vi "Initialization_T_B_ver1.0.vi"(1 "output cluster":T1={"Main Sweep"=0, "Steps Config:"={"total points:"=0, "Step Delay (s)"=0.0, "Ini Delay (s)"=0.0, "# of steps:"=0}, "Temperature Control (ITC 503):"={"GPIB ADR"=0, "Change Heater?"={"Heater?"=FALSE, "Heater"=0}, "Change Temp?"={"Change T?"=FALSE, "Set T (K)"=0.0}, "Cluster"={"Heat Auto?"=FALSE, "Manual Heat?"=FALSE, "Heater (%)"=0.0}, "Change PID?"={"Change PID?"=FALSE, "P"=0.0, "I"=0.0, "D"=0.0}, "Change Para?"=FALSE, "Sensor"=1}, "Temperature Control (LS 340):"={"GPIB ADR"=0, "From (K)"=0.0, "To (K)"=0.0, "Rate (K/min)"=0.0, "Delta T (0.08K)"=0.0, "Temp. Header"="", "T Display Control"={"Ch B"=FALSE, "Ch C"=FALSE, "Ch D"=FALSE}}, "Magnet Control (IPS 120-10)"={"Action"=0, "Standby (s)"=0.0, "Heater on (s)"=0.0, "Sweep Setup "=[], "GPIB ADR"=0, "Change Para?"=FALSE}, "Keithley 6221 :"=[], "Measuring Instruments : "=[], "Lock-In SR7265 :"=[], "Deascription of \nthis measurement"="", "Instruments Config:"=[]} {"Main Sweep" items=["Time", "DC Current", "Delta Current", "Pulse Delta Current", "Sine Current", "Lock-in Vosc"]; "Temperature Control (ITC 503):"."Sensor" items=["T2", "T3"]; "Magnet Control (IPS 120-10)"."Action" items=["Hold", "To Set point", "To Zero", "Clamp"]; "Keithley 6221 :"."Sweep Mode" items=["Linear", "Log", "Exp", "Inverse", "Manual"]}, 5 "Measure with H/T sweep?":bool, 6 "error in (no error)":errorcluster, 7 "First run?":bool, 8 "Last run?":bool, 9 "B Field Display Tex Array":refnum<vi>[](array[refnum]), 10 "Temp. Display Ref Array":refnum<vi>[](array[refnum])) -> (0 "error out":errorcluster, 2 "output cluster 2":T1={"Main Sweep"=0, "Steps Config:"={"total points:"=0, "Step Delay (s)"=0.0, "Ini Delay (s)"=0.0, "# of steps:"=0}, "Temperature Control (ITC 503):"={"GPIB ADR"=0, "Change Heater?"={"Heater?"=FALSE, "Heater"=0}, "Change Temp?"={"Change T?"=FALSE, "Set T (K)"=0.0}, "Cluster"={"Heat Auto?"=FALSE, "Manual Heat?"=FALSE, "Heater (%)"=0.0}, "Change PID?"={"Change PID?"=FALSE, "P"=0.0, "I"=0.0, "D"=0.0}, "Change Para?"=FALSE, "Sensor"=1}, "Temperature Control (LS 340):"={"GPIB ADR"=0, "From (K)"=0.0, "To (K)"=0.0, "Rate (K/min)"=0.0, "Delta T (0.08K)"=0.0, "Temp. Header"="", "T Display Control"={"Ch B"=FALSE, "Ch C"=FALSE, "Ch D"=FALSE}}, "Magnet Control (IPS 120-10)"={"Action"=0, "Standby (s)"=0.0, "Heater on (s)"=0.0, "Sweep Setup "=[], "GPIB ADR"=0, "Change Para?"=FALSE}, "Keithley 6221 :"=[], "Measuring Instruments : "=[], "Lock-In SR7265 :"=[], "Deascription of \nthis measurement"="", "Instruments Config:"=[]} {"Main Sweep" items=["Time", "DC Current", "Delta Current", "Pulse Delta Current", "Sine Current", "Lock-in Vosc"]; "Temperature Control (ITC 503):"."Sensor" items=["T2", "T3"]; "Magnet Control (IPS 120-10)"."Action" items=["Hold", "To Set point", "To Zero", "Clamp"]; "Keithley 6221 :"."Sweep Mode" items=["Linear", "Log", "Exp", "Inverse", "Manual"]}, 3 "Title Array":string[](array[string]), 4 "Comments String":string)   [LabVIEW 2011]
doc: "Initialize the temperature (LS336)"
panel:
  out "BField Display Cluster":cluster{"B":dbl} {"B" min=0.0 format="%_5f"}
  out "B Set Pt (T)":dbl format="%_5g"
  out "B Rate (T/min)":dbl format="%_5g"
  out "Temp Graph 2":dbl[][](graph)=[[348.0650696299951, 348.0650696299951, 348.0650696299951, 348.0650696299951, 348.0650696299951, 348.0650696299951, 348.0650696299951, 348.0650696299951, 348.0650696299951, 348.0650696299951, 348.0650696299951, 348.0650696299951, 348.0650696299951, 348.0650696299951, 348.0650696299951], [349.0, 349.0, 349.0, 349.0, 349.0, 349.0, 349.0, 349.0, 349.0, 349.0, 349.0, 349.0, 349.0, 349.0, 349.0], [347.994, 347.998, 348.007, 348.013, 348.031, 348.047, 348.071, 348.073, 348.076, 348.088, 348.106, 348.11, 348.113, 348.121, 348.128], [349.08, 349.08, 349.08, 349.08, 349.08, 349.08, 349.08, 349.08, 349.08, 349.08, 349.08, 349.08, 349.08, 349.08, 349.08], [348.92, 348.92, 348.92, 348.92, 348.92, 348.92, 348.92, 348.92, 348.92, 348.92, 348.92, 348.92, 348.92, 348.92, 348.92]]
  out "StartTime":u32
  in  "Skip":bool
  out "Time 2":string
  in  "Timeout (min)":u32=30
  out "Reach to set pt?":bool
  out "T Rate (K/min)":dbl format="%_5g"
  out "T Set Pt (K)":dbl format="%_5g"
  out "Temp Display Cluster":cluster{"RMS T:":dbl, "T STD":dbl, "T":dbl} {"T STD" min=0.0 format="%8.4f"; "T" min=0.0 format="%_5f"; "RMS T:" format="%_5g"}
  out "Temp Graph":dbl[][](graph)=[[348.0650696299951, 348.0650696299951, 348.0650696299951, 348.0650696299951, 348.0650696299951, 348.0650696299951, 348.0650696299951, 348.0650696299951, 348.0650696299951, 348.0650696299951, 348.0650696299951, 348.0650696299951, 348.0650696299951, 348.0650696299951, 348.0650696299951], [349.0, 349.0, 349.0, 349.0, 349.0, 349.0, 349.0, 349.0, 349.0, 349.0, 349.0, 349.0, 349.0, 349.0, 349.0], [347.994, 347.998, 348.007, 348.013, 348.031, 348.047, 348.071, 348.073, 348.076, 348.088, 348.106, 348.11, 348.113, 348.121, 348.128], [349.08, 349.08, 349.08, 349.08, 349.08, 349.08, 349.08, 349.08, 349.08, 349.08, 349.08, 349.08, 349.08, 349.08, 349.08], [348.92, 348.92, 348.92, 348.92, 348.92, 348.92, 348.92, 348.92, 348.92, 348.92, 348.92, 348.92, 348.92, 348.92, 348.92]]
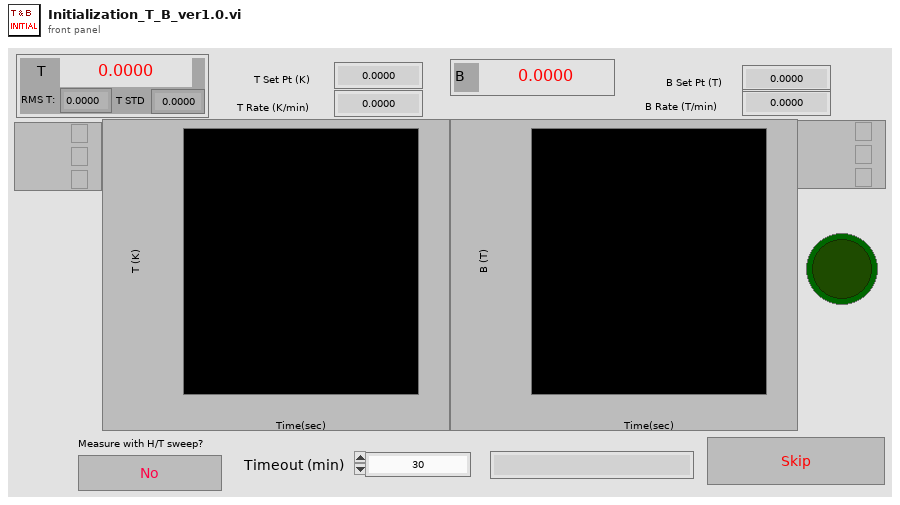
[diagram p1: front panel]
types:
  T1 = cluster{"Main Sweep":u8, "Steps Config:":cluster{"total points:":u32, "Step Delay (s)":dbl, "Ini Delay (s)":dbl, "# of steps:":u32}, "Temperature Control (ITC 503):":cluster{"GPIB ADR":u16, "Change Heater?":cluster{"Heater?":bool, "Heater":u8}, "Change Temp?":cluster{"Change T?":bool, "Set T (K)":dbl}, "Cluster":cluster{"Heat Auto?":bool, "Manual Heat?":bool, "Heater (%)":dbl}, "Change PID?":cluster{"Change PID?":bool, "P":dbl, "I":dbl, "D":dbl}, "Change Para?":bool, "Sensor":u16}, "Temperature Control (LS 340):":cluster{"GPIB ADR":u16, "From (K)":dbl, "To (K)":dbl, "Rate (K/min)":dbl, "Delta T (0.08K)":dbl, "Temp. Header":string, "T Display Control":cluster{"Ch B":bool, "Ch C":bool, "Ch D":bool}}, "Magnet Control (IPS 120-10)":cluster{"Action":u16, "Standby (s)":dbl, "Heater on (s)":dbl, "Sweep Setup ":cluster{"Set Point (T)":dbl, "Set Rate(T/min)":dbl, "Hold(min)":dbl}[], "GPIB ADR":u16, "Change Para?":bool}, "Keithley 6221 :":cluster{"Delta mode":bool, "Const I":bool, "Pulse Delta mode":bool, "Sine Wave Mode":bool, "From I_HI (A)":dbl, "From I (A)":dbl, "I_LO (A)":dbl, "From I_H (A)":dbl, "I_L (A)":dbl, "Freq (Hz)":dbl, "From I_Sin (A)":dbl, "DC Offset (A)":dbl, "Delay Time (s)":dbl, "Pulse Width (s)":dbl, "Delay (s)":dbl, "To I (A)":dbl, "ASymmetric?":bool, "To I_HI (A)":dbl, "To I_H (A)":dbl, "To I_Sin (A)":dbl, "GPIB ADR":u16, "Sweep Mode":u8, "Delta Unit":string, "2182A range (V)":dbl, "6221 Compliance (V)":dbl}[], "Measuring Instruments : ":cluster{"GPIB Bus":dbl, "GPIB Addr":dbl, "Instrument":enum16{"None", "HP34401DMM", "Lockin 7265", "HP3456/7A", "HP3478A", "HP3325FG", "Keithley2182A"}, "Instru Header":string}[], "Lock-In SR7265 :":cluster{"GPIB ADR":u16, "From":dbl, "To":dbl, "Header(;)":string, "Sweep Mode":u8}[], "Deascription of \nthis measurement":string, "Instruments Config:":string[][]}
  T2 = cluster{"GPIB ADR":u16, "Change Heater?":cluster{"Heater?":bool, "Heater":u8}, "Change Temp?":cluster{"Change T?":bool, "Set T (K)":dbl}, "Cluster":cluster{"Heat Auto?":bool, "Manual Heat?":bool, "Heater (%)":dbl}, "Change PID?":cluster{"Change PID?":bool, "P":dbl, "I":dbl, "D":dbl}, "Change Para?":bool, "Sensor":u16}
  T3 = cluster{"GPIB ADR":u16, "From (K)":dbl, "To (K)":dbl, "Rate (K/min)":dbl, "Delta T (0.08K)":dbl, "Temp. Header":string, "T Display Control":cluster{"Ch B":bool, "Ch C":bool, "Ch D":bool}}
  T4 = cluster{"Action":u16, "Standby (s)":dbl, "Heater on (s)":dbl, "Sweep Setup ":cluster{"Set Point (T)":dbl, "Set Rate(T/min)":dbl, "Hold(min)":dbl}[], "GPIB ADR":u16, "Change Para?":bool}
  T5 = cluster{"RMS":dbl, "STD":dbl, "Current value":dbl}
  T6 = cluster{"Com Port":i32, "ISOBUS Address":i32, "GPIB Address":i16, "Communication":enum16{"RS232", "ISOBUS", "GPIB", "Gateway"}}
  T7 = cluster{"GPIB ADR":u16, "Change Heater?":cluster{"Change Heater?":bool, "Heater":u8}, "Change Temp?":cluster{"Change Temp?":bool, "Set Temp (K)":dbl}, "Cluster":cluster{"Heat Auto?":bool, "Manual Heat?":bool, "Heater Manual (%)":dbl}, "Change PID?":cluster{"Change PID?":bool, "Proportional":dbl, "Integral":dbl, "Derivative":dbl}, "Change Para?":bool, "ITC503 Control Sensor":u16}
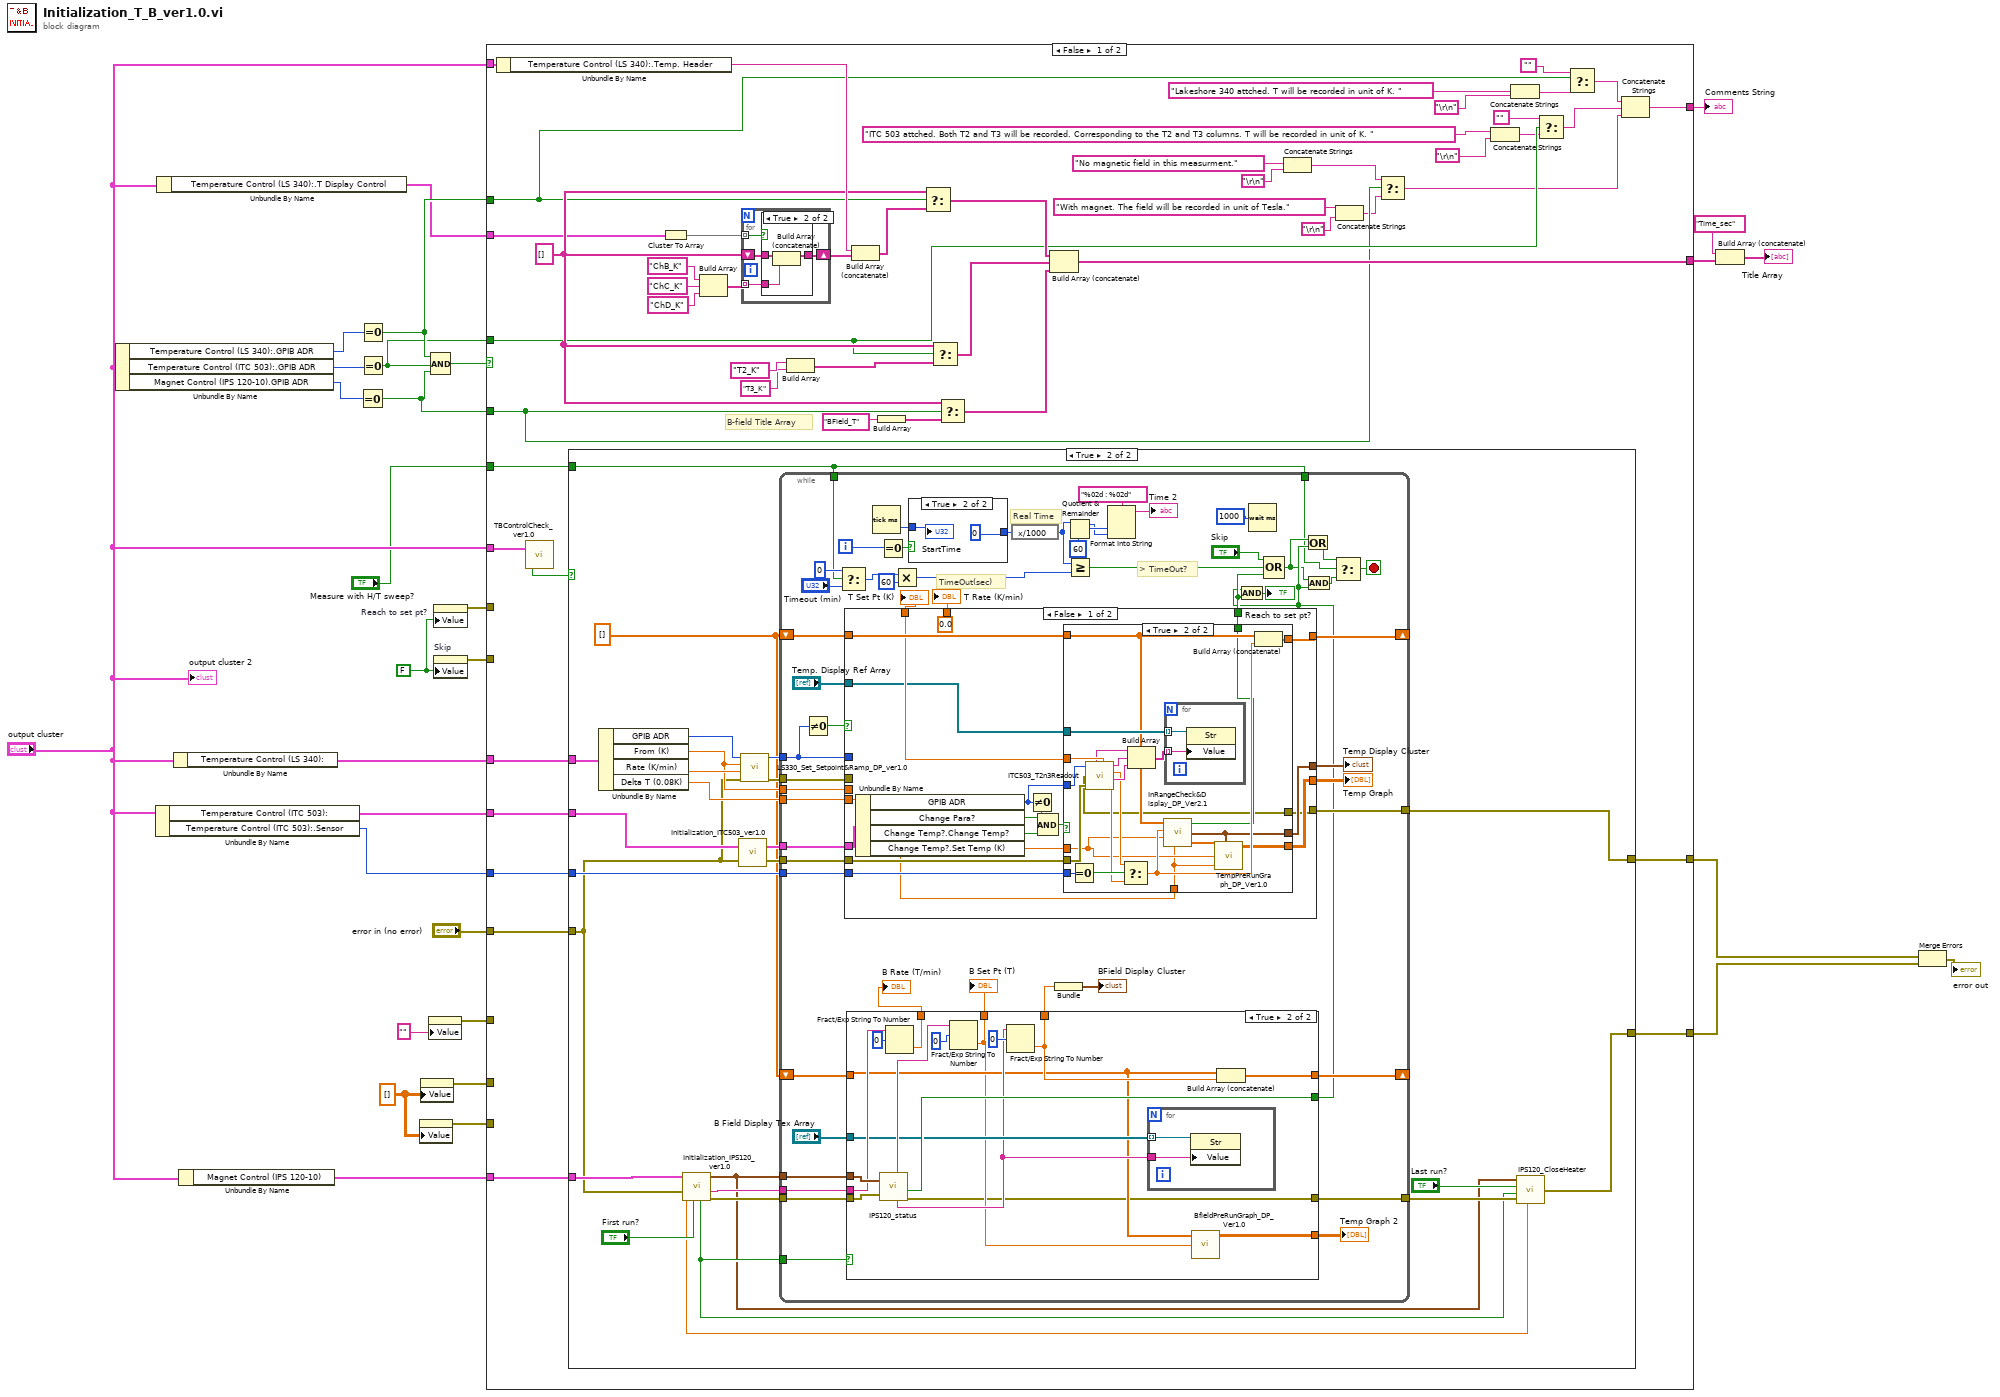
[diagram p0: block diagram]
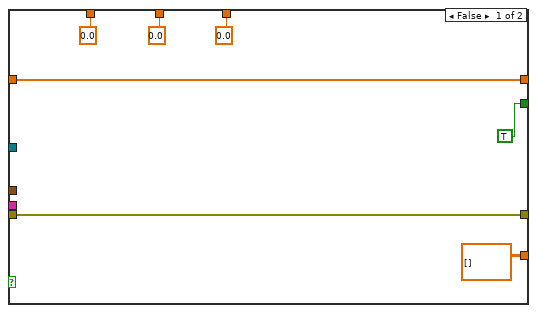
[diagram p3: hidden frame]
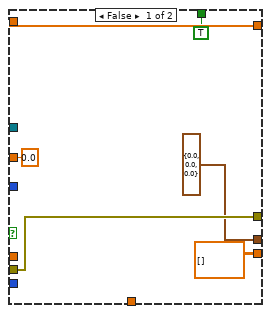
[diagram p4: hidden frame]
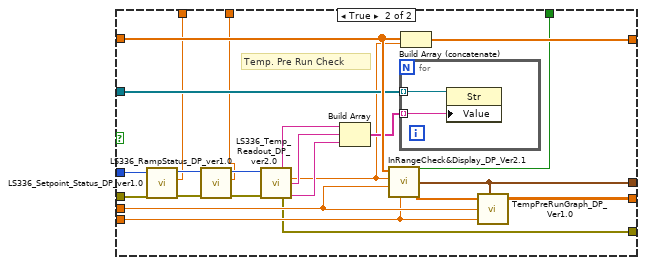
[diagram p5: hidden frame]
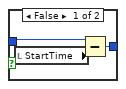
[diagram p6: hidden frame]
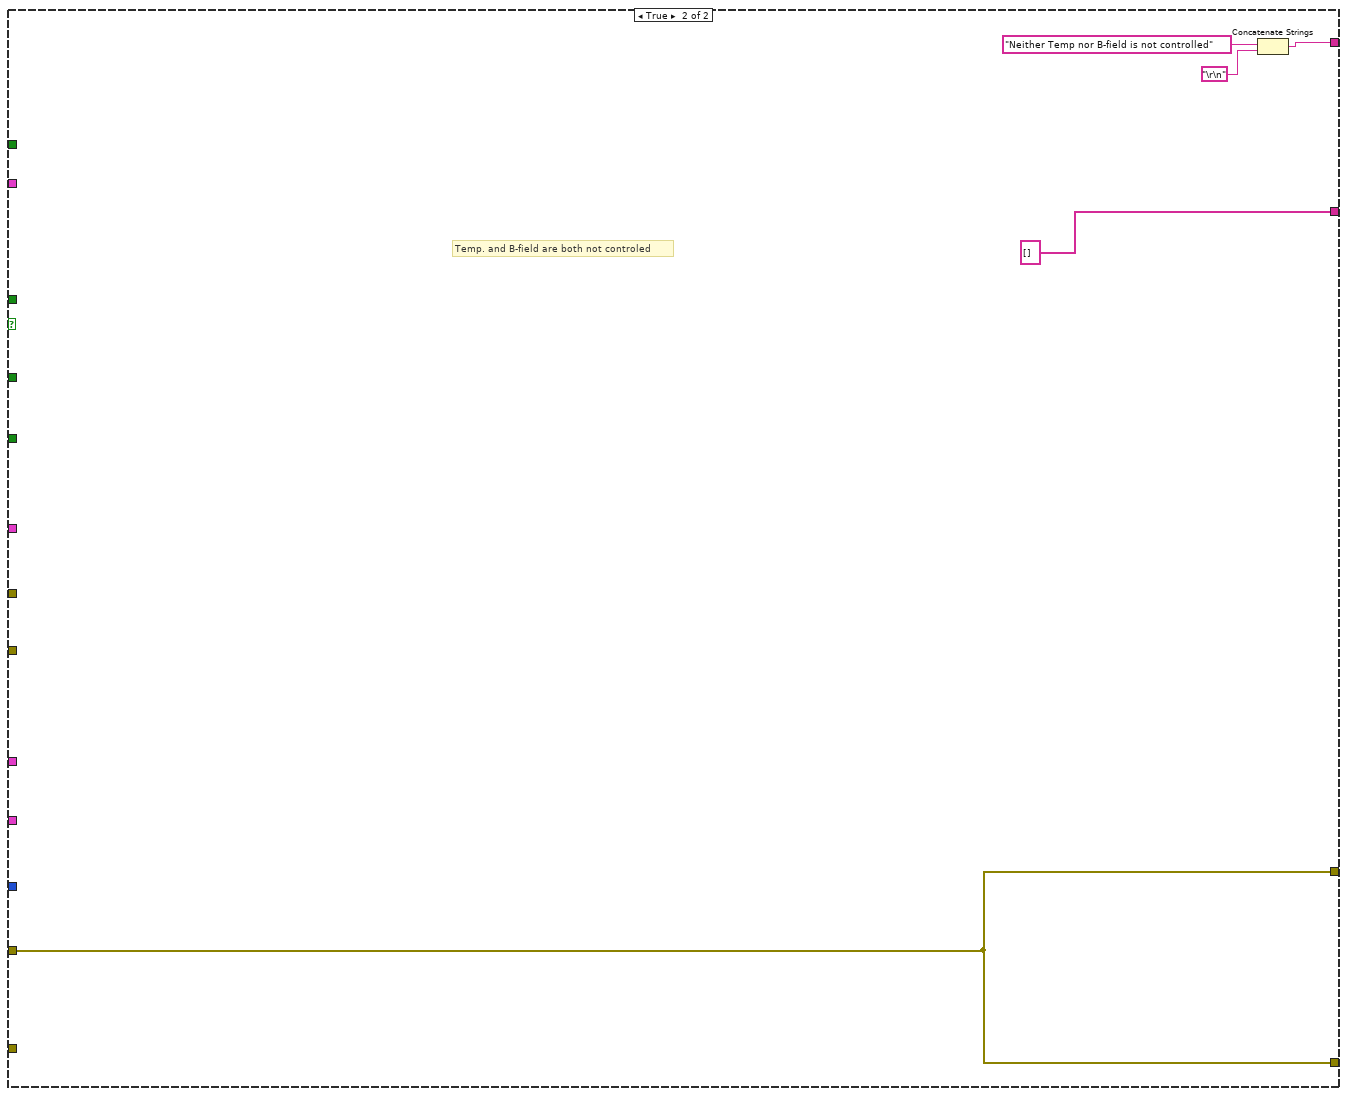
[diagram p8: hidden frame]
diagram:
  w4 = FALSE ("Skip")
  w11 = dbl[][] []
  n1 = Unbundle By Name("output cluster") -> ("Temperature Control (LS 340):.GPIB ADR"=w30:u16, "Temperature Control (ITC 503):.GPIB ADR"=w29:u16, "Magnet Control (IPS 120-10).GPIB ADR"=w28:u16)
  n2 = Unbundle By Name("output cluster") -> ("Temperature Control (ITC 503):"=w15:T2, "Temperature Control (ITC 503):.Sensor"=w2:u16)
  n3 = Unbundle By Name("output cluster") -> ("Temperature Control (LS 340):.T Display Control"=w12:cluster{"Ch B":bool, "Ch C":bool, "Ch D":bool})
  n4 = Unbundle By Name("output cluster") -> ("Temperature Control (LS 340):"=w16:T3)
  n5 = Unbundle By Name("output cluster") -> ("Magnet Control (IPS 120-10)"=w14:T4)
  n6 = Equal To 0?(x=w28) -> (x = 0?=w17:bool)
  n7 = Equal To 0?(x=w30) -> (x = 0?=w19:bool)
  n8 = Equal To 0?(x=w29) -> (x = 0?=w18:bool)
  n9 = property on="Temp Graph 2" class="WFGraph (strict)"("Value"=w11) -> (error out=w9:errorcluster)  [unwired: 2 in, 1 out]
  n10 = property on="Temp Graph" class="WFGraph (strict)"("Value"=w11) -> (error out=w10:errorcluster)  [unwired: 2 in, 1 out]
  n11 = property on="Time 2" class="Str"("Value"="" ("Time 2")) -> (error out=w7:errorcluster)  [unwired: 2 in, 1 out]
  n12 = Compound Arithmetic op=AND(w19, w18, w17) -> (w27:bool)
  n13 = property on="Reach to set pt?" class="Bool (strict)"("Value"=w4) -> (error out=w5:errorcluster)  [unwired: 2 in, 1 out]
  n14 = property on="Skip" class="Bool (strict)"("Value"=w4) -> (error out=w6:errorcluster)  [unwired: 2 in, 1 out]
  n15 = case shown="False" w27 {
    tunnel: [w71 string[] []] -> w25
    tunnel: "error in (no error)" -> [w60 w280]
    tunnel: [w59 w280] -> w21
    tunnel: [w58 w280] -> w20
    tunnel: "output cluster" -> [w76 _]
    tunnel: w19 -> [w53 _]
    tunnel: w18 -> [w48 _]
    tunnel: w17 -> [w40 _]
    tunnel: "output cluster" -> [w62 _]
    tunnel: w16 -> [w57 _]
    tunnel: w15 -> [w56 _]
    tunnel: w14 -> [w55 _]
    tunnel: [w34 w277] -> w13
    tunnel: w12 -> [w33 _]
    tunnel: w2 -> [w32 _]
    tunnel: w10 -> [_ _]
    tunnel: w9 -> [_ _]
    tunnel: w7 -> [_ _]
    tunnel: w6 -> [_ _]
    tunnel: w5 -> [_ _]
    tunnel: "Measure with H/T sweep?" -> [w31 _]
    frame False {
      w66 = string[] []
      # "B-field Title Array"
      n16 = Unbundle By Name(w76) -> ("Temperature Control (LS 340):.Temp. Header"=w74:string)
      n17 = call "TBControlCheck_ver1.0.vi"("output cluster"=w62) -> ("T&B Setting Change?"=w61:bool)  [unwired: 3 out]
      n18 = case shown="True" w61 {
        tunnel: w60 -> [w82 w94]
        tunnel: [w82 w98] -> w59
        tunnel: [w82 w90] -> w58
        tunnel: w57 -> [_ w106]
        tunnel: w56 -> [_ w107]
        tunnel: w55 -> [_ w95]
        tunnel: w32 -> [_ w96]
        tunnel: w31 -> [_ w83]
        frame False {
        }
        frame True {
          w91 = dbl[] []
          n19 = Unbundle By Name(w106) -> ("GPIB ADR"=w105:u16, "From (K)"=w101:dbl, "Rate (K/min)"=w104:dbl, "Delta T (0.08K)"=w100:dbl)
          n20 = call "Initialization_IPS120_ver1.0.vi"("Magnet Control (IPS 120-10)"=w95, "error in"=w94, "First run?"="First run?") -> ("Hold(min)"=w84:dbl, "B field Change?"=w88:bool, "output cluster"=w86:T6, "Rate"=w92:string, "error out"=w93:errorcluster)  [unwired: 3 out]
          n21 = call "Initialization_ITC503_ver1.0.vi"("error in"=w94, "Temperature Control (ITC 503):"=w107) -> ("error out"=w99:errorcluster, "Temperature Control (ITC 503): 2"=w97:T7)
          n22 = call "LS330_Set_Setpoint&Ramp_DP_ver1.0.vi"("error in"=w94, "Ramping rate (0-100 K/min; 1.0)"=w104, "Setpoint (2-400 K)"=w101, "GPIB ADR (19)"=w105) -> ("error out"=w102:errorcluster, "dump GPIB ADR"=w103:i16)  [unwired: 6 in]
          n23 = while {
            tunnel: w103 -> [w145]
            tunnel: w102 -> [w144]
            shift-right: [w146] -> _
            shift-left: w91 -> [w147]
            tunnel: w101 -> [w143]
            tunnel: w100 -> [w142]
            tunnel: w99 -> [w135]
            tunnel: [w134] -> w98
            tunnel: w97 -> [w133]
            tunnel: w96 -> [w132]
            tunnel: w88 -> [w131]
            tunnel: w86 -> [w130]
            tunnel: w93 -> [w129]
            tunnel: w92 -> [w128]
            shift-right: [w122] -> _
            shift-left: w91 -> [w123]
            tunnel: [w119] -> w89
            tunnel: w83 -> [w112]
            tunnel: w83 -> [w108]
            i -> [w151]
            stop <- w113 stop-if-true
            # "Real Time"
            # "> TimeOut?"
            # "TimeOut(sec)"
            n24 = Not Equal To 0?(x=w145) -> (x != 0?=w148:bool)
            n25 = Select(t=u32 0, s=w108, f="Timeout (min)") -> (s? t:f=w110:u32)
            n26 = case shown="False" w148 {
              tunnel: w147 -> [w207 w251]
              tunnel: [w206 w261] -> w146
              tunnel: w145 -> [_ w260]
              tunnel: w144 -> [_ w259]
              tunnel: w143 -> [_ w249]
              tunnel: w142 -> [w194 w248]
              tunnel: [w191 w247] -> w118
              tunnel: "Temp. Display Ref Array" -> [w196 w245]
              tunnel: [w190 w244] -> w134
              tunnel: [w198 w242] -> w139
              tunnel: [0.0 ("Ramp Rate") w241] -> w138
              tunnel: [w192 w240] -> w137
              tunnel: [w193 w239] -> w136
              tunnel: w135 -> [w208 _]
              tunnel: w133 -> [w205 _]
              tunnel: w132 -> [w195 _]
              frame False {
                n27 = Unbundle By Name(w205) -> ("GPIB ADR"=w200:u16, "Change Para?"=w202:bool, "Change Temp?.Change Temp?"=w201:bool, "Change Temp?.Set Temp (K)"=w199:dbl)
                n28 = Not Equal To 0?(x=w200) -> (x != 0?=w203:bool)
                n29 = Compound Arithmetic op=AND(w203, w202, w201) -> (w204:bool)
                n30 = case shown="True" w204 {
                  tunnel: w208 -> [w212 w236]
                  tunnel: w207 -> [w214 w223]
                  tunnel: [w214 w235] -> w206
                  tunnel: w200 -> [_ w234]
                  tunnel: w199 -> [_ w218]
                  tunnel: [0.0 ("Set T") w233] -> w198
                  tunnel: w196 -> [_ w229]
                  tunnel: w195 -> [_ w227]
                  tunnel: w194 -> [_ w217]
                  tunnel: [T5 {"RMS"=0.0, "STD"=0.0, "Current value"=0.0} ("Display Cluster") w220] -> w193
                  tunnel: [dbl[][] [] ("Temp Graph") w219] -> w192
                  tunnel: [TRUE ("Reach to set pt?") w216] -> w191
                  tunnel: [w212 w215] -> w190
                  frame False {
                  }
                  frame True {
                    n31 = Equal To 0?(x=w227) -> (x = 0?=w226:bool)
                    n32 = call "ITC503_T2n3Readout.vi"("GPIB Address"=w234, "error in"=w236) -> ("error out"=w215:errorcluster, "Sensor T1"=w232:string, "Set T"=w233:dbl, "Sensor T2"=w231:string, "T2"=w225:dbl, "Sensor T3"=w230:string, "T3"=w224:dbl)  [unwired: 2 out]
                    n33 = Select(t=w225, s=w226, f=w224) -> (s? t:f=w222:dbl)
                    n34 = Build Array(w232, w231, w230) -> (w228:string[])
                    n35 = call "InRangeCheck&Display_DP_Ver2.1.vi"("Delta range>0"=w217, "Set Point"=w218, "Current value"=w222, "Data Array In"=w223) -> ("Data Array Out"=w221:dbl[], "Display Cluster"=w220:T5, "Reach to set pt?"=w216:bool)  [unwired: 4 in]
                    n36 = for {
                      tunnel: w228 -> [w237] mode=indexing
                      tunnel: w229 -> [w238] mode=indexing
                      n37 = property class="Str"(reference=w238, "Value"=w237) -> ()  [unwired: 1 in, 2 out]
                    }
                    n38 = call "TempPreRunGraph_DP_Ver1.0.vi"("T Array"=w221, "Temp Display Cluster (Need RMS)"=w220, "Set Pt"=w218, "Delta T"=w217) -> ("Temp Graph"=w219:dbl[][])  [unwired: 3 in]
                    n39 = Build Array (concatenate)(w223, w222) -> (w235:dbl[])
                  }
                }
              }
              frame True {
                # "Temp. Pre Run Check"
                n40 = call "LS336_Setpoint_Status_DP_ver1.0.vi"("error in"=w259, "GPIB ADR (18)"=w260) -> ("error out"=w257:errorcluster, "Setpoint"=w242:dbl, "dump GPIB ADR"=w258:i16)  [unwired: 2 in, 1 out]
                n41 = call "LS336_RampStatus_DP_ver1.0.vi"("GPIB ADR (18)"=w258, "error in"=w257) -> ("dump GPIB ADR"=w256:i16, "Ramp Rate"=w241:dbl, "error out"=w255:errorcluster)  [unwired: 2 in, 3 out]
                n42 = call "LS336_Temp_Readout_DP_ver2.0.vi"("GPIB ADR (18)"=w256, "error in"=w255) -> (2:"Sensor A (K)"=w243:dbl, 3:"Sensor A (K)"=w254:string, "Sensor B (K)"=w253:string, "error out"=w244:errorcluster, "Sensor C (K)"=w252:string)  [unwired: 4 in, 5 out]
                n43 = Build Array(w254, w253, w252) -> (w246:string[])
                n44 = call "InRangeCheck&Display_DP_Ver2.1.vi"("Delta range>0"=w248, "Set Point"=w249, "Current value"=w243, "Data Array In"=w251) -> ("Data Array Out"=w250:dbl[], "Display Cluster"=w239:T5, "Reach to set pt?"=w247:bool)  [unwired: 4 in]
                n45 = for {
                  tunnel: w246 -> [w262] mode=indexing
                  tunnel: w245 -> [w263] mode=indexing
                  n46 = property class="Str"(reference=w263, "Value"=w262) -> ()  [unwired: 1 in, 2 out]
                }
                n47 = Build Array (concatenate)(w251, w243) -> (w261:dbl[])
                n48 = call "TempPreRunGraph_DP_Ver1.0.vi"("T Array"=w250, "Temp Display Cluster (Need RMS)"=w239, "Set Pt"=w249, "Delta T"=w248) -> ("Temp Graph"=w240:dbl[][])  [unwired: 3 in]
              }
            }
            "T Set Pt (K)" <- w139
            "T Rate (K/min)" <- w138
            "Temp Display Cluster" <- w136
            "Temp Graph" <- w137
            n49 = case shown="True" w131 {
              tunnel: [TRUE ("B field change stop") w185] -> w117
              tunnel: w130 -> [_ w187]
              tunnel: w129 -> [w164 w186]
              tunnel: w128 -> [_ w184]
              tunnel: [0.0 w182] -> w127
              tunnel: [0.0 w173] -> w126
              tunnel: [0.0 w177] -> w125
              tunnel: w123 -> [w169 w174]
              tunnel: [w169 w178] -> w122
              tunnel: "B Field Display Tex Array" -> [_ w176]
              tunnel: [dbl[][] [] ("BField Graph") w172] -> w120
              tunnel: [w164 w171] -> w119
              frame False {
              }
              frame True {
                n50 = call "IPS120_status.vi"("Address"=w187, "error in"=w186) -> ("Set point"=w180:string, "Real Field"=w175:string, "Arrive"=w185:bool, "error out"=w171:errorcluster)  [unwired: 2 out]
                n51 = Fract/Exp String To Number(string=w184, offset=0) -> (number=w182:dbl)  [unwired: 2 in, 1 out]
                n52 = Fract/Exp String To Number(string=w180, offset=0) -> (number=w173:dbl)  [unwired: 2 in, 1 out]
                n53 = Fract/Exp String To Number(string=w175, offset=0) -> (number=w177:dbl)  [unwired: 2 in, 1 out]
                n54 = for {
                  tunnel: w175 -> [w188]
                  tunnel: w176 -> [w189] mode=indexing
                  n55 = property class="Str"(reference=w189, "Value"=w188) -> ()  [unwired: 1 in, 2 out]
                }
                n56 = call "BfieldPreRunGraph_DP_Ver1.0.vi"("B Array"=w174, "Set Pt"=w173) -> ("BField Graph"=w172:dbl[][])  [unwired: 5 in]
                n57 = Build Array (concatenate)(w174, w177) -> (w178:dbl[])
              }
            }
            "B Set Pt (T)" <- w126
            "B Rate (T/min)" <- w127
            "Temp Graph 2" <- w120
            n58 = Tick Count (ms)() -> (millisecond timer value=w160:u32)
            n59 = Equal To 0?(x=w151) -> (x = 0?=w161:bool)
            n60 = Multiply(x=w110, y=u32 60) -> (x*y=w154:u32)
            n61 = case shown="True" w161 {
              tunnel: w160 -> [w265 w268]
              tunnel: [w266 0] -> w162
              frame False {
                n62 = local read "StartTime"() -> (w264:u32)
                n63 = Subtract(x=w265, y=w264) -> (x-y=w266:u32)
              }
              frame True {
                "StartTime" <- w268
              }
            }
            n64 = expression code="x/1000"(w162) -> (w156:u32)
            n65 = Bundle(w125) -> (→"BField Display Cluster":cluster{dbl})  [unwired: 1 in]
            n66 = Quotient & Remainder(x=w156, y=u32 60) -> (x-y*floor(x/y)=w158:u32, floor(x/y)=w159:u32)
            n67 = Greater Or Equal?(x=w156, y=w154) -> (x >= y?=w153:bool)
            n68 = Format Into String(format string="%02d : %02d", w159, w158) -> (resulting string=→"Time 2":string)  [unwired: 2 in, 1 out]
            n69 = And(x=w117, y=w118) -> (x .and. y?=→"Reach to set pt?":bool)
            n70 = Wait (ms)(milliseconds to wait=u32 1000) -> ()  [unwired: 1 out]
            n71 = Compound Arithmetic op=OR("Skip", w153, w118) -> (w116:bool)
            n72 = Or(x=w116, y=w117) -> (x .or. y?=w114:bool)
            n73 = And(x=w116, y=w117) -> (x .and. y?=w115:bool)
            n74 = Select(t=w114, s=w112, f=w115) -> (s? t:f=w113:bool)
          }
          n75 = call "IPS120_CloseHeater.vi"("Instrument address (in)"=w86, "Last run?"="Last run?", "B field Change?"=w88, "error in"=w89, "Hold(min)"=w84) -> ("error out"=w90:errorcluster)
        }
      }
      n76 = Cluster To Array(cluster=w33) -> (array=w81:bool[])
      n77 = Build Array("ChB_K" ("f"), "ChC_K" ("f"), "ChD_K" ("f")) -> (w77:string[])
      n78 = for {
        tunnel: w81 -> [w272] mode=indexing
        shift-right: [w269] -> w75
        shift-left: w66 -> [w270]
        tunnel: w77 -> [w271] mode=indexing
        n79 = case shown="True" w272 {
          tunnel: w271 -> [_ w276]
          tunnel: w270 -> [w273 w275]
          tunnel: [w273 w274] -> w269
          frame False {
          }
          frame True {
            n80 = Build Array (concatenate)(w275, w276) -> (w274:string[])
          }
        }
      }
      n81 = Build Array("T2_K" ("f"), "T3_K" ("f")) -> (w68:string[])
      n82 = Build Array (concatenate)(w74, w75) -> (w73:string[])
      n83 = Build Array("BField_T" ("f")) -> (w64:string[])
      n84 = Select(t=w66, s=w53, f=w73) -> (s? t:f=w72:string[])
      n85 = Select(t=w66, s=w48, f=w68) -> (s? t:f=w67:string[])
      n86 = Select(t=w66, s=w40, f=w64) -> (s? t:f=w63:string[])
      n87 = Build Array (concatenate)(w72, w67, w63) -> (w71:string[])
      n88 = Concatenate Strings("No magnetic field in this measurment.", "\r\n") -> (w39:string)
      n89 = Concatenate Strings("With magnet. The field will be recorded in unit of Tesla.", "\r\n") -> (w38:string)
      n90 = Select(t=w39, s=w40, f=w38) -> (s? t:f=w35:string)
      n91 = Concatenate Strings("ITC 503 attched. Both T2 and T3 will be recorded. Corresponding to the T2 and T3 columns. T will be recorded in unit of K. ", "\r\n") -> (w46:string)
      n92 = Concatenate Strings("Lakeshore 340 attched. T will be recorded in unit of K. ", "\r\n") -> (w51:string)
      n93 = Select(t="", s=w48, f=w46) -> (s? t:f=w36:string)
      n94 = Select(t="", s=w53, f=w51) -> (s? t:f=w37:string)
      n95 = Concatenate Strings(w37, w36, w35) -> (w34:string)
    }
    frame True {
      # "Temp. and B-field are both not controled"
      n96 = Concatenate Strings("Neither Temp nor B-field is not controlled", "\r\n") -> (w277:string)
    }
  }
  "Comments String" <- w13
  n97 = Build Array (concatenate)("Time_sec", w25) -> (→"Title Array":string[])
  n98 = Merge Errors(w21, w20) -> (→"error out":errorcluster)
  "output cluster 2" <- "output cluster"
